vi "Drivetrain Trapezoidal Control.vi"(10 "Axes":T1) -> ()   [LabVIEW 2017]
uses:
  Common Code/Gamepads/Axes Cluster.ctl
  Common Code/Trapezoidal States.ctl
  Robot Global Data.vi
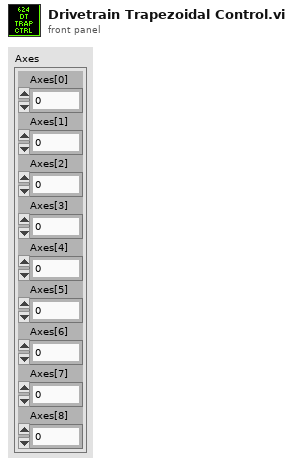
[diagram p1: front panel]
types:
  T1 = typedef "Axes Cluster.ctl" = cluster{"Axes[0]":dbl, "Axes[1]":dbl, "Axes[2]":dbl, "Axes[3]":dbl, "Axes[4]":dbl, "Axes[5]":dbl, "Axes[6]":dbl, "Axes[7]":dbl, "Axes[8]":dbl}
  T2 = typedef "Trapezoidal States.ctl" = enum16{"Feed Forward", "Feed Backwards", "Cruise", "Shift Feed Forward", "Shift Feed Backwards", "Shift Cruise", "Idle"}
  T3 = typedef "Drivetrain Command Cluster.ctl" = cluster{"Y Power":dbl, "Turn Power":dbl, "Drivetrain Mode":T4, "2nd Gear":bool, "Y Min Output":dbl, "Y Max Output":dbl, "X Min Output":dbl, "X Max Output":dbl, "Heading Target":dbl, "Distance Target":dbl, "Brake?":bool, "Zero Gyro":bool, "Trapezoidal States":T2}
  T4 = typedef "Drivetrain Mode.ctl" = enum16{"Trapezoidal Motion", "Manual", "Gyro Steer", "PID Drive", "Distance Drive", "Autonomous"}
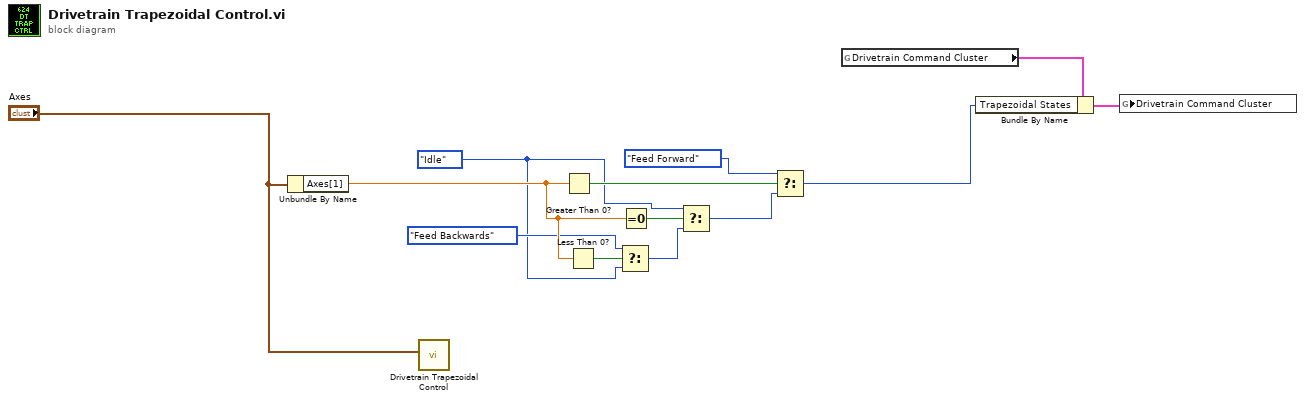
[diagram p0: block diagram]
diagram:
  w2 = Trapezoidal_States."Idle" ("Trapezoidal States")
  n1 = Unbundle By Name("Axes") -> ("Axes[1]"=w6:dbl)
  n2 = call "Drivetrain Trapezoidal Control.vi"("Axes"="Axes") -> ()  [unwired: 11 in]
  n3 = Greater Than 0?(x=w6) -> (x > 0?=w10:bool)
  n4 = Less Than 0?(x=w6) -> (x < 0?=w5:bool)
  n5 = Select(t=Trapezoidal_States."Feed Backwards" ("Trapezoidal States"), s=w5, f=w2) -> (s? t:f=w3:T2)
  n6 = Equal To 0?(x=w6) -> (x = 0?=w8:bool)
  n7 = Select(t=w2, s=w8, f=w3) -> (s? t:f=w7:T2)
  n8 = Select(t=Trapezoidal_States."Feed Forward" ("Trapezoidal States"), s=w10, f=w7) -> (s? t:f=w1:T2)
  n9 = global read "Robot Global Data.vi" "Drivetrain Command Cluster"() -> (w13:T3)
  n10 = Bundle By Name(cluster=w13, "Trapezoidal States"=w1) -> (w12:T3)
  n11 = global write "Robot Global Data.vi" "Drivetrain Command Cluster"(w12) -> ()
